vi "type to wait boolean.vi"(11 "类型":T1) -> (3 "簇":T2)   [LabVIEW 2019, in "User lib.lvlib"]
uses:
  User lib.lvlib
  ctl/set type.ctl
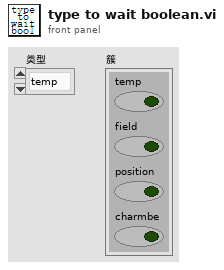
[diagram p1: front panel]
types:
  T1 = typedef "set type.ctl" = enum16{"temp", "field", "position", "gating", "current", "PZT", "time"}
  T2 = cluster{"temp":bool, "field":bool, "position":bool, "charmbe":bool}
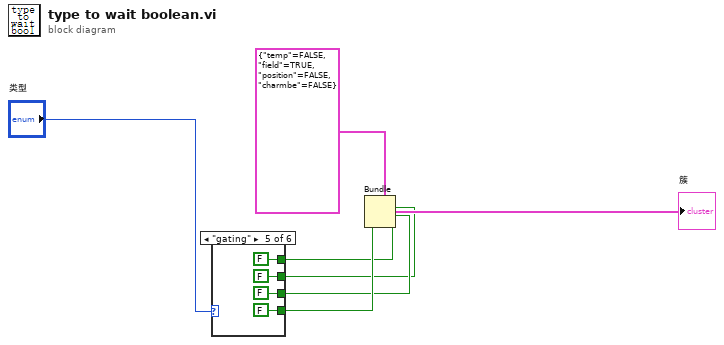
[diagram p0: block diagram]
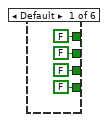
[diagram p2: hidden frame]
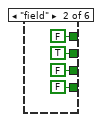
[diagram p3: hidden frame]
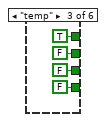
[diagram p4: hidden frame]
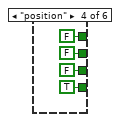
[diagram p5: hidden frame]
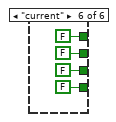
[diagram p6: hidden frame]
diagram:
  n1 = case shown="\"gating\"" "类型" {
    tunnel: [FALSE FALSE TRUE FALSE FALSE FALSE] -> w2
    tunnel: [FALSE TRUE FALSE FALSE FALSE FALSE] -> w3
    tunnel: [FALSE FALSE FALSE TRUE FALSE FALSE] -> w5
    tunnel: [FALSE FALSE FALSE FALSE FALSE FALSE] -> w4
    frame Default {
    }
    frame "field" {
    }
    frame "temp" {
    }
    frame "position" {
    }
    frame "gating" {
    }
    frame "current" {
    }
  }
  n2 = Bundle(cluster=T2 {"temp"=FALSE, "field"=TRUE, "position"=FALSE, "charmbe"=FALSE}, "temp"=w2, "field"=w3, "position"=w4, "charmbe"=w5) -> (→"簇":T2)
